vi "Configure All.vi"(1 "RT Data in":T1={"Device ref"=0, "Scan Period (uSec)"=10000, "Device Channels"={"Status"={"BD Refs"=[], "Length"=0, "FIFO Index"=0, "Data"=[]}, "Command"={"BD Refs"=[], "Data"=[], "Length"=0, "FIFO Index"=0}}, "Local Chassis"=[], "EtherCAT Masters"=[], "Async"={"Status"=refnum, "Command"=refnum, "Input FIFO"=refnum, "Input FIFO buffer"=[], "Output FIFO"=refnum, "Output FIFO buffer"=[], "Async VI Ref"=refnum}, "ECAT Reconfig"={"Reconfig Module Found"=FALSE, "VI Ref"=refnum, "Status"=refnum}, "Device Error"={"status"=FALSE, "code"=0, "source"=""}, "DeviceName"="", "PCLSync?"=FALSE} {"Device Channels"."Status"."BD Refs"."Data Reference" format="%.0x"; "Device Channels"."Command"."BD Refs"."Data Reference" format="%.0x"; "Local Chassis"."FPGA"."VS ref" format="%.0x"; "Local Chassis"."RSI Modules"."VS ref" format="%.0x"; "Local Chassis"."VS ref" format="%.0x"; "Device ref" format="%.0x"; "EtherCAT Masters"."VS ref" format="%.0x"; "EtherCAT Masters"."EtherCAT Slaves"."FPGA"."VS ref" format="%.0x"; "EtherCAT Masters"."EtherCAT Slaves"."RSI Modules"."VS ref" format="%.0x"; "EtherCAT Masters"."EtherCAT Slaves"."VS ref" format="%.0x"}) -> (0 "RT Data out":T1={"Device ref"=0, "Scan Period (uSec)"=10000, "Device Channels"={"Status"={"BD Refs"=[], "Length"=0, "FIFO Index"=0, "Data"=[]}, "Command"={"BD Refs"=[], "Data"=[], "Length"=0, "FIFO Index"=0}}, "Local Chassis"=[], "EtherCAT Masters"=[], "Async"={"Status"=refnum, "Command"=refnum, "Input FIFO"=refnum, "Input FIFO buffer"=[], "Output FIFO"=refnum, "Output FIFO buffer"=[], "Async VI Ref"=refnum}, "ECAT Reconfig"={"Reconfig Module Found"=FALSE, "VI Ref"=refnum, "Status"=refnum}, "Device Error"={"status"=FALSE, "code"=0, "source"=""}, "DeviceName"="", "PCLSync?"=FALSE} {"Device Channels"."Status"."BD Refs"."Data Reference" format="%.0x"; "Device Channels"."Command"."BD Refs"."Data Reference" format="%.0x"; "Local Chassis"."FPGA"."VS ref" format="%.0x"; "Local Chassis"."RSI Modules"."VS ref" format="%.0x"; "Local Chassis"."VS ref" format="%.0x"; "Device ref" format="%.0x"; "EtherCAT Masters"."VS ref" format="%.0x"; "EtherCAT Masters"."EtherCAT Slaves"."FPGA"."VS ref" format="%.0x"; "EtherCAT Masters"."EtherCAT Slaves"."RSI Modules"."VS ref" format="%.0x"; "EtherCAT Masters"."EtherCAT Slaves"."VS ref" format="%.0x"})   [LabVIEW 2016, in "Scan Engine Custom Device.lvlib"]
uses:
  Scan Engine Custom Device.lvlib
  Modules.lvlibp/RSI Module/RSI Module.lvclass
  Type Defs/ECAT Module Reconfig.ctl
  <vilib>/NI Veristand/Custom Device API/Custom Device Item Ref.ctl
  <vilib>/NI Veristand/Custom Device API/Custom Device API.lvlib
  <vilib>/NI Veristand/Custom Device API/Data Reference.ctl
  <vilib>/NI Veristand/Custom Device API/Block Data Reference.ctl
  Type Defs/Input Data.ctl
  Type Defs/Output Data.ctl
  Type Defs/RSI Module Data.ctl
  Type Defs/FPGA Data.ctl
  Type Defs/Local Chassis Data.ctl
  Type Defs/EtherCAT Slave Data.ctl
  Type Defs/EtherCAT Master Data.ctl
  Type Defs/RT Data.ctl
  Modules.lvlibp/RSI Module/Channel Type.ctl
  Type Defs/Async Command.ctl
  Type Defs/Async Status.ctl
  Type Defs/Async State.ctl
  Type Defs/UDV Data Type.ctl
  Type Defs/FXP Config.ctl
  Type Defs/UDV Data.ctl
  Modules.lvlibp/RSI Module/Module Models.ctl
  Type Defs/Module Config Data.ctl
  Type Defs/Async Data.ctl
  Type Defs/ECAT Reconfig State.ctl
  Type Defs/ECAT Reconfig Status.ctl
  Type Defs/ECAT Reconfig Data.ctl
  Type Defs/Device Channels.ctl
  Type Defs/Mixed IO.ctl
  Type Defs/Open Module IOVs.ctl
  Type Defs/Mod Size Indexes.ctl
types:
  T1 = typedef "Scan Engine Custom Device.lvlib/RT Data.ctl" = cluster{"Device ref":T2, "Scan Period (uSec)":u32, "Device Channels":T3, "Local Chassis":T8[], "EtherCAT Masters":T20[], "Async":T22, "ECAT Reconfig":T23, "Device Error":errorcluster, "DeviceName":string, "PCLSync?":bool}
  T2 = typedef "Custom Device API.lvlib/Custom Device Item Ref.ctl" = u64
  T3 = typedef "Scan Engine Custom Device.lvlib/Device Channels.ctl" = cluster{"Status":T4, "Command":T7}
  T4 = typedef "Scan Engine Custom Device.lvlib/Output Data.ctl" = cluster{"BD Refs":T5[], "Length":i32, "FIFO Index":i32, "Data":dbl[]}
  T5 = typedef "Custom Device API.lvlib/Block Data Reference.ctl" = cluster{"Data Reference":T6, "Offset":u64, "Length":u64}
  T6 = typedef "Custom Device API.lvlib/Data Reference.ctl" = i32
  T7 = typedef "Scan Engine Custom Device.lvlib/Input Data.ctl" = cluster{"BD Refs":T5[], "Data":dbl[], "Length":i32, "FIFO Index":i32}
  T8 = typedef "Scan Engine Custom Device.lvlib/Local Chassis Data.ctl" = cluster{"VS ref":T2, "RSI Modules":T9[], "FPGA":T15[], "Input Mod Size Idxs":T19, "Output Modules":i32[], "MixedIO Mod Size Idxs":T19}
  T9 = typedef "Scan Engine Custom Device.lvlib/RSI Module Data.ctl" = cluster{"VS ref":T2, "IOV ref":refnum<k21>, "Open Mod refs":T10, "Module DVR":refnum<data-value>, "Slot":u32, "Model":T11, "Channel Type":T12, "EtherCAT?":bool, "CDInput Data":T7, "CDOutput Data":T4, "Module Config Data":T13, "Mixed IO":T14}
  T10 = typedef "Scan Engine Custom Device.lvlib/Open Module IOVs.ctl" = cluster{"Analog Read":refnum<k21>, "Digital Read":refnum<k21>, "Analog Write":refnum<k21>, "Digital Write":refnum<k21>}
  T11 = typedef "Modules.lvlibp/RSI Module.lvclass/Module Models.ctl" = enum16{"Empty", "NI 9201", "NI 9203", "NI 9205", "NI 9206", "NI 9207", "NI 9208", "NI 9211", "NI 9213", "NI 9214", "NI 9215", "NI 9217", "NI 9219", "NI 9221", "NI 9225", "NI 9227", "NI 9229", "NI 9233", "NI 9234", "NI 9235", "NI 9236", "NI 9237", "NI 9239", "NI 9263", "NI 9264", "NI 9265", "NI 9269", "NI 9375", "NI 9401", "NI 9402", "NI 9403", "NI 9411", "NI 9421", "NI 9422", "NI 9423", "NI 9425", "NI 9426", "NI 9435", "NI 9472", "NI 9474", "NI 9475", "NI 9476", "NI 9477", "NI 9478", "NI 9481", "NI 9482", "NI 9485"}
  T12 = typedef "Modules.lvlibp/RSI Module.lvclass/Channel Type.ctl" = enum16{"Analog", "Digital"}
  T13 = typedef "Scan Engine Custom Device.lvlib/Module Config Data.ctl" = cluster{"Configurable?":bool, "Config Block Data Refs":T5[], "Config Data DVR":refnum<data-value>, "Previous Values":dbl[], "Local Reconfig VI Ref":refnum<vi>}
  T14 = typedef "Scan Engine Custom Device.lvlib/Mixed IO.ctl" = cluster{"Input Channel Indices":i32[], "Input Buffer":dbl[]}
  T15 = typedef "Scan Engine Custom Device.lvlib/FPGA Data.ctl" = cluster{"VS ref":T2, "IOV ref":refnum<k21>, "FPGA Target":enum16{"Local", "EtherCAT"}, "Product Code":u32, "Bitfile Signature":string, "Bitfile Path (RT)":path, "FPGA Session":u32, "Input Data":T7, "Output Data":T4, "UDVs":cluster{"From FPGA":T16[], "To FPGA":T16[]}}
  T16 = typedef "Scan Engine Custom Device.lvlib/UDV Data.ctl" = cluster{"VS ref":T2, "IOV Ref":refnum<k21>, "Name":string, "UDV Data Type":T17, "Supported Type?":bool, "FXP Config":T18, "FXP VI Ref":refnum<vi>}
  T17 = typedef "Scan Engine Custom Device.lvlib/UDV Data Type.ctl" = enum16{"Boolean", "Fixed Point", "Int8", "Int16", "Int32", "Int64", "U32 Bit Field", "UInt8", "UInt16", "UInt32", "UInt64", "Other"}
  T18 = typedef "Scan Engine Custom Device.lvlib/FXP Config.ctl" = cluster{"signed":bool, "size":u32, "integersize":i32}
  T19 = typedef "Scan Engine Custom Device.lvlib/Mod Size Indexes.ctl" = cluster{"4":i32[], "8":i32[], "16":i32[], "32":i32[], "other":i32[]}
  T20 = typedef "Scan Engine Custom Device.lvlib/EtherCAT Master Data.ctl" = cluster{"VS ref":T2, "IOV ref":refnum<k21>, "Master ID":u32, "Cyclic Data Bandwidth":u32, "EtherCAT Slaves":T21[]}
  T21 = typedef "Scan Engine Custom Device.lvlib/EtherCAT Slave Data.ctl" = cluster{"VS ref":T2, "IOV ref":refnum<k21>, "Position Address":u16, "RSI Modules":T9[], "FPGA":T15[], "Input Mod Size Idxs":T19, "Output Modules":i32[], "MixedIO Mod Size Idxs":T19}
  T22 = typedef "Scan Engine Custom Device.lvlib/Async Data.ctl" = cluster{"Status":refnum<queue>, "Command":refnum<queue>, "Input FIFO":refnum<k33>, "Input FIFO buffer":dbl[], "Output FIFO":refnum<k33>, "Output FIFO buffer":dbl[], "Async VI Ref":refnum<vi>}
  T23 = typedef "Scan Engine Custom Device.lvlib/ECAT Reconfig Data.ctl" = cluster{"Reconfig Module Found":bool, "VI Ref":refnum<vi>, "Status":refnum<queue>}
  T24 = typedef "Scan Engine Custom Device.lvlib/ECAT Module Reconfig.ctl" = cluster{"Module DVR":refnum<data-value>, "IOV ref":refnum<k21>, "Config Data DVR":refnum<data-value>}
  T25 = typedef "Scan Engine Custom Device.lvlib/RSI Module Data.ctl" = cluster{"VS ref":T2, "IOV ref":refnum<k21>, "Module DVR":refnum<data-value>, "Slot":u32, "Model":T11, "Channel Type":T12, "EtherCAT?":bool, "Input Data":T7, "Output Data":T4, "Module Config Data":T13, "Mixed IO":T14}
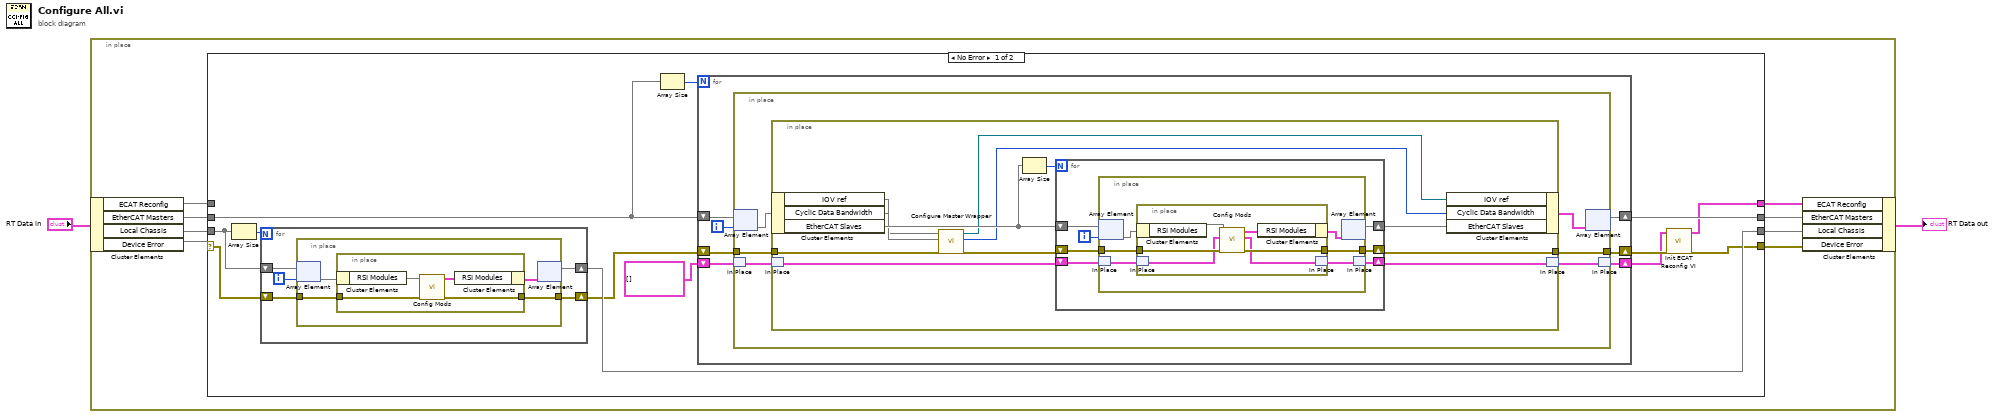
[diagram p0: block diagram]
diagram:
  n1 = in-place {
    n2 = in-place-cluster #1("RT Data in") -> ("ECAT Reconfig"=w3, "EtherCAT Masters"=w9, "Local Chassis"=w8, "Device Error"=w10)
    n3 = case shown="No Error" w10 {
      selector: w10 -> [w18 w84]
      tunnel: [w13 w84] -> w7
      tunnel: w9 -> [w22 w82]
      tunnel: w8 -> [w19 w83]
      tunnel: [w17 w83] -> w6
      tunnel: [w21 w82] -> w5
      tunnel: [w11 w81] -> w4
      tunnel: w3 -> [_ w81]
      frame No Error {
        n4 = Array Size(array=w19) -> (size(s)=w20:i32)
        n5 = for {
          N: w20 -> [_]
          shift-right: [w24] -> w17
          shift-left: w19 -> [w28]
          shift-right: [w25] -> w16
          shift-left: w18 -> [w26]
          i -> [w27]
          n6 = in-place {
            in-place-border: w26 -> [w30]
            in-place-border: [w29] -> w25
            n7 = in-place-array #2(w28, w27) -> (w32)
            n8 = in-place {
              in-place-border: w30 -> [w34]
              in-place-border: [w33] -> w29
              n9 = in-place-cluster #3(w32) -> ("RSI Modules"=w36)
              n10 = call "Config Mods.vi"("error in (no error)"=w34, "RSI Modules in"=w36) -> ("error out"=w33:errorcluster, "RSI Modules out"=w35:T25[])  [unwired: 7 in, 1 out]
              n11 = in-place-cluster #3("RSI Modules"=w35) -> (w31:cluster{})
            }
            n12 = in-place-array #2(w31) -> (w24)  [unwired: 1 out]
          }
        }
        n13 = Array Size(array=w22) -> (size(s)=w23:i32)
        n14 = for {
          N: w23 -> [_]
          shift-right: [w40] -> w14
          shift-left: w16 -> [w41]
          shift-right: [w39] -> w21
          shift-left: w22 -> [w43]
          shift-right: [w37] -> w12
          shift-left: T24[] [] -> [w38]
          i -> [w42]
          n15 = in-place {
            in-place-border: w41 -> [w48]
            in-place-border: [w47] -> w40
            n16 = in-place-array #4(w43, w42) -> (w49)
            n17 = in-place-match #5(w38) -> (w45:T24[])
            n18 = in-place {
              in-place-border: w48 -> [w55]
              in-place-border: [w59] -> w47
              n19 = in-place-cluster #6(w49) -> ("IOV ref"=w53, "Cyclic Data Bandwidth"=w54, "EtherCAT Slaves"=w61)
              n20 = in-place-match #7(w45) -> (w57:T24[])
              n21 = call "Configure Master Wrapper.vi"("error in"=w55, "Cyclic Data Bandwidth"=w54, "IOV ref in"=w53) -> ("error out"=w52:errorcluster, "Cyclic Data Bandwidth out"=w51:u32, "IOV ref out"=w50:refnum<k21>)  [unwired: 6 in]
              n22 = Array Size(array=w61) -> (size(s)=w60:i32)
              n23 = for {
                N: w60 -> [_]
                shift-right: [w65] -> w59
                shift-left: w52 -> [w66]
                shift-right: [w64] -> w58
                shift-left: w61 -> [w68]
                shift-right: [w62] -> w56
                shift-left: w57 -> [w63]
                i -> [w67]
                n24 = in-place {
                  in-place-border: w66 -> [w73]
                  in-place-border: [w72] -> w65
                  n25 = in-place-array #8(w68, w67) -> (w74)
                  n26 = in-place-match #9(w63) -> (w70:T24[])
                  n27 = in-place {
                    in-place-border: w73 -> [w78]
                    in-place-border: [w77] -> w72
                    n28 = in-place-cluster #10(w74) -> ("RSI Modules"=w80)
                    n29 = in-place-match #11(w70) -> (w76:T24[])
                    n30 = call "Config Mods.vi"("error in (no error)"=w78, "ECAT Mod Reconfig in"=w76, "RSI Modules in"=w80) -> ("error out"=w77:errorcluster, "ECAT Mod Reconfig out"=w75:T24[], "RSI Modules out"=w79:T25[])  [unwired: 6 in]
                    n31 = in-place-cluster #10("RSI Modules"=w79) -> (w71:cluster{})
                    n32 = in-place-match #11(w75) -> (w69:T24[])
                  }
                  n33 = in-place-array #8(w71) -> (w64)  [unwired: 1 out]
                  n34 = in-place-match #9(w69) -> (w62:T24[])
                }
              }
              n35 = in-place-cluster #6("IOV ref"=w50, "Cyclic Data Bandwidth"=w51, "EtherCAT Slaves"=w58) -> (w46:cluster{})
              n36 = in-place-match #7(w56) -> (w44:T24[])
            }
            n37 = in-place-array #4(w46) -> (w39)  [unwired: 1 out]
            n38 = in-place-match #5(w44) -> (w37:T24[])
          }
        }
        n39 = call "Init ECAT Reconfig VI.vi"("error in (no error)"=w14, "ECAT Modules"=w12) -> ("error out"=w13:errorcluster, "ECAT Reconfig out"=w11:T23)  [unwired: 8 in]
      }
      frame Error {
      }
    }
    n40 = in-place-cluster #1("ECAT Reconfig"=w4, "EtherCAT Masters"=w5, "Local Chassis"=w6, "Device Error"=w7) -> (→"RT Data out":cluster{})
  }
